vi "Write Properties Pane.vi"(8 "error in (no error)":errorcluster, 10 "Properties Pane":refnum<vi>, 11 "Imager Handler in":refnum<class "Imager Handler.lvclass">) -> (0 "error out":errorcluster, 3 "Imager Handler out":refnum<class "Imager Handler.lvclass">)   [LabVIEW 2016, in "Imager Handler.lvclass"]
uses:
  Imager Handler.lvclass
  Imager Handler.lvclass/Imager Handler.ctl
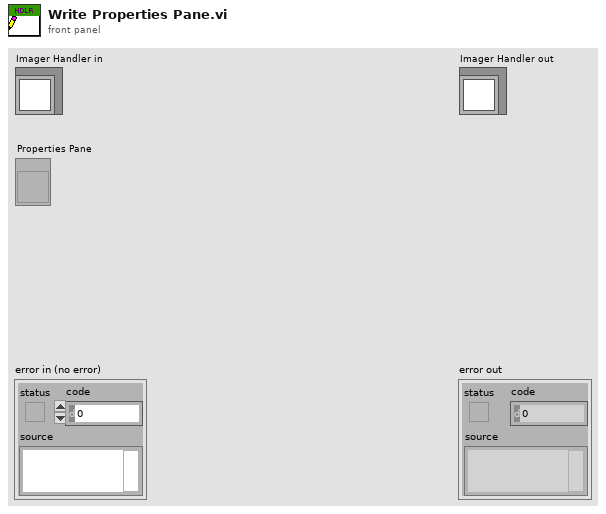
[diagram p1: front panel]
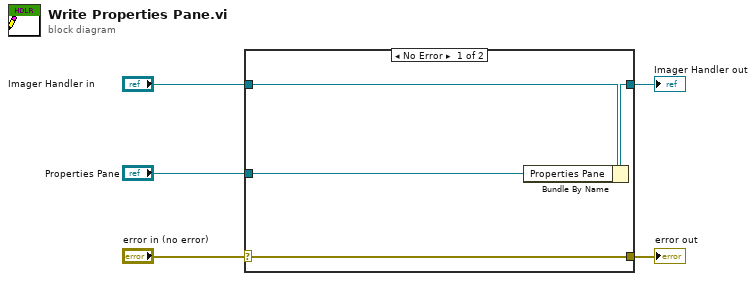
[diagram p0: block diagram]
diagram:
  n1 = case shown="No Error" "error in (no error)" {
    selector: "error in (no error)" -> [w9 w10]
    tunnel: [w9 w10] -> w4
    tunnel: [w7 w11] -> w2
    tunnel: "Imager Handler in" -> [w8 w11]
    tunnel: "Properties Pane" -> [w6 _]
    frame No Error {
      n2 = Bundle By Name(cluster=w8, "Properties Pane"=w6) -> (w7:refnum<class "Imager Handler.lvclass">)
    }
    frame Error {
    }
  }
  "error out" <- w4
  "Imager Handler out" <- w2
